vi "AlGaInPAs_ext_v00.vi"(2 "Debug Mode":bool, 3 "Elapsed Time(s)":dbl, 4 "State":enum16{"Edit", "Start", "Run", "End", "Idle"}(ring), 5 "Argument List In":string[](array[string])) -> (0 "Status Out":string, 1 "Argument List Out":string[](array[string]))   [LabVIEW 2011]
panel:
  in  "Pbub Prep":bool caption="Pre-run"
  out "Pbub Prep var":bool
  out "Pbub?":bool
  in  "Pbub Flow":dbl caption="P bubbler Flow (0-100 sccm)" format="%.2f"
  in  "Pbub Run":bool caption="Run"
  out "GAMFC3 var":dbl=100.0 caption="R3 (0-1000 sscm)" format="%.1f"
  out "GAMFC2 var":dbl=10.0 caption="R2 (0-100 sscm)" format="%.2f"
  out "GAMFC1 var":dbl caption="R1 (0-10 sscm)" format="%.2f"
  out "Ga Flow var":dbl caption="Ga Flow (0-10 sscm)" format="%.4f"
  out "In Prep var":bool
  out "Ga Prep var":bool
  out "Al Prep var":bool
  out "PH3 Prep var":bool
  out "AsH3 Prep var":bool
  out "prep_done":bool
  out "run started":bool
  out "first":bool=TRUE
  out "total time":dbl
  out "is OK?":bool
  out "AsH3?":bool
  out "PH3?":bool
  out "In?":bool
  out "Ga?":bool
  out "Al?":bool
  in  "AsH3 Prep":bool caption="Pre-run"
  in  "PH3 Prep":bool caption="Pre-run"
  in  "In Prep":bool caption="Pre-run"
  in  "prep_time":dbl caption="pre-run time (s)"
  in  "Al Prep":bool caption="Pre-run"
  in  "AsH3 Run":bool caption="Run"
  in  "AsH3 Flow":dbl caption="AsH3 Flow (0-10 sccm)" format="%.2f"
  in  "PH3 Flow":dbl caption="PH3 Flow (0-100 sccm)" format="%.2f"
  in  "PH3 Run":bool caption="Run"
  in  "In Flow":dbl caption="In Flow (0-100 sscm)" format="%.2f"
  in  "In Run":bool caption="Run"
  in  "Al Run":bool caption="Run"
  in  "Al Flow":dbl caption="Al Flow (0-100 sscm)" format="%.2f"
  in  "Cancel":bool
  in  "OK":bool
  out "tTotal(s) 2":dbl
  in  "Ga Tab Control":enum32{"Page 1", "Page 2", "Page 3"}(tab)
  in  "Ga Dilution":bool caption="Dilute"
  in  "Ga Run":bool caption="Run"
  in  "Ga Prep":bool caption="Pre-run"
  out "Ga Flow val":dbl=1.0 caption="Ga Flow (0-10 sscm)" format="%.4f"
  in  "Ga Flow set":dbl caption="Ga Flow (0-10 sscm)" format="%.4f"
  out "GAMFC1 val":dbl caption="R1 (0-10 sscm)" format="%.4f"
  out "GAMFC3 val":dbl=100.0 caption="R3 (0-1000 sscm)" format="%.1f"
  out "GAMFC2 val":dbl=10.0 caption="R2 (0-100 sscm)" format="%.2f"
  in  "GAMFC1 set":dbl=1.0 caption="R1 (0-10 sscm)" format="%.2f"
  in  "GAMFC2 set":dbl=10.0 caption="R2 (0-100 sscm)" format="%.2f"
  in  "GAMFC3 set":dbl=100.0 caption="R3 (0-1000 sscm)" format="%.1f"
  in  "Ga Calculated":u16(ring)=1 caption="Calculated" items=["Ga flow", "MFC1", "MFC2", "MFC3"]
  # "Add pre-run time to run time in editor."
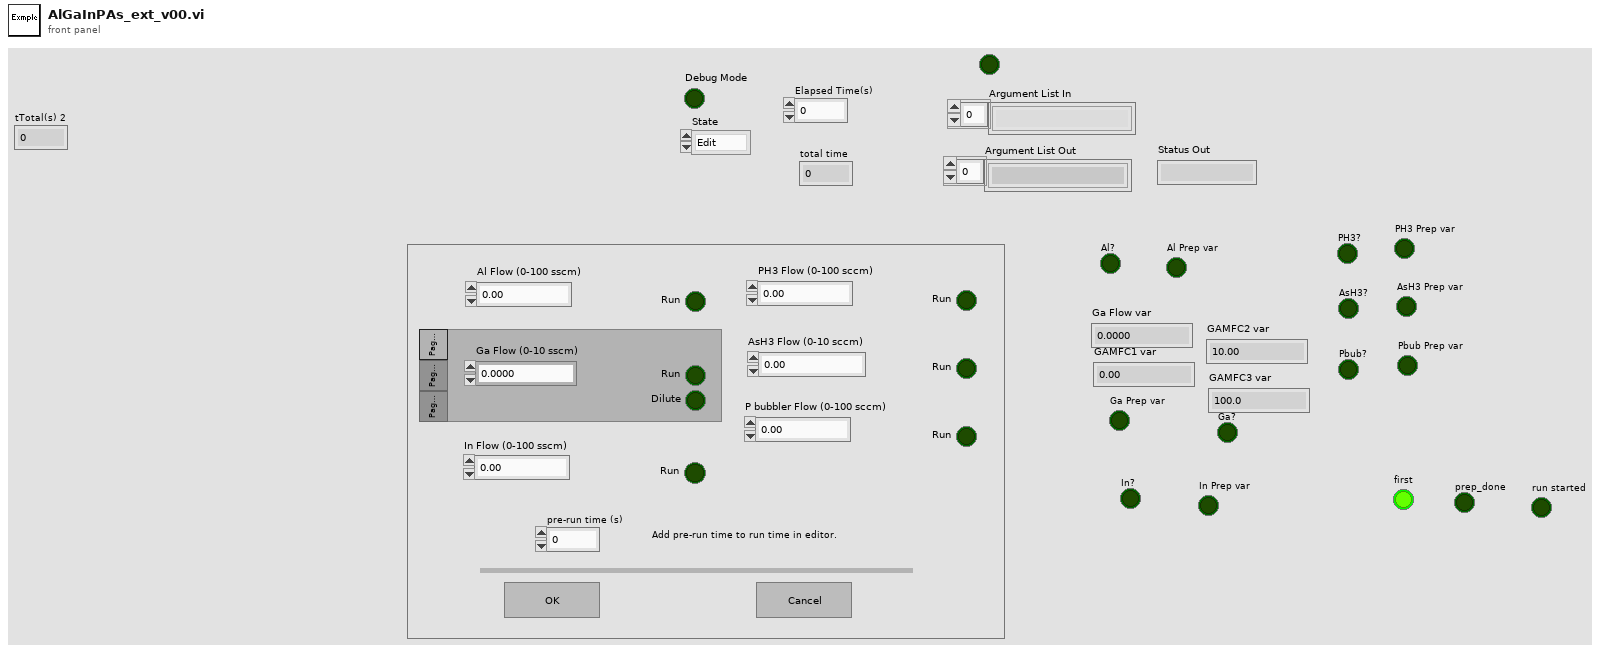
[diagram p1: front panel]
types:
  T1 = enum16{"Discrete", "Continuous", "Instantaneous", "Finite"}
  T2 = enum32{"Invalid", "Default", "Floating", "Floating/Auto-Hide", "Modal"}
  T3 = cluster{"Ga val":bool, "MFC1 val":bool, "MFC2 val":bool, "MFC3 val":bool, "Ga set":bool, "MFC1 set":bool, "MFC2 set":bool, "MFC3 set":bool}
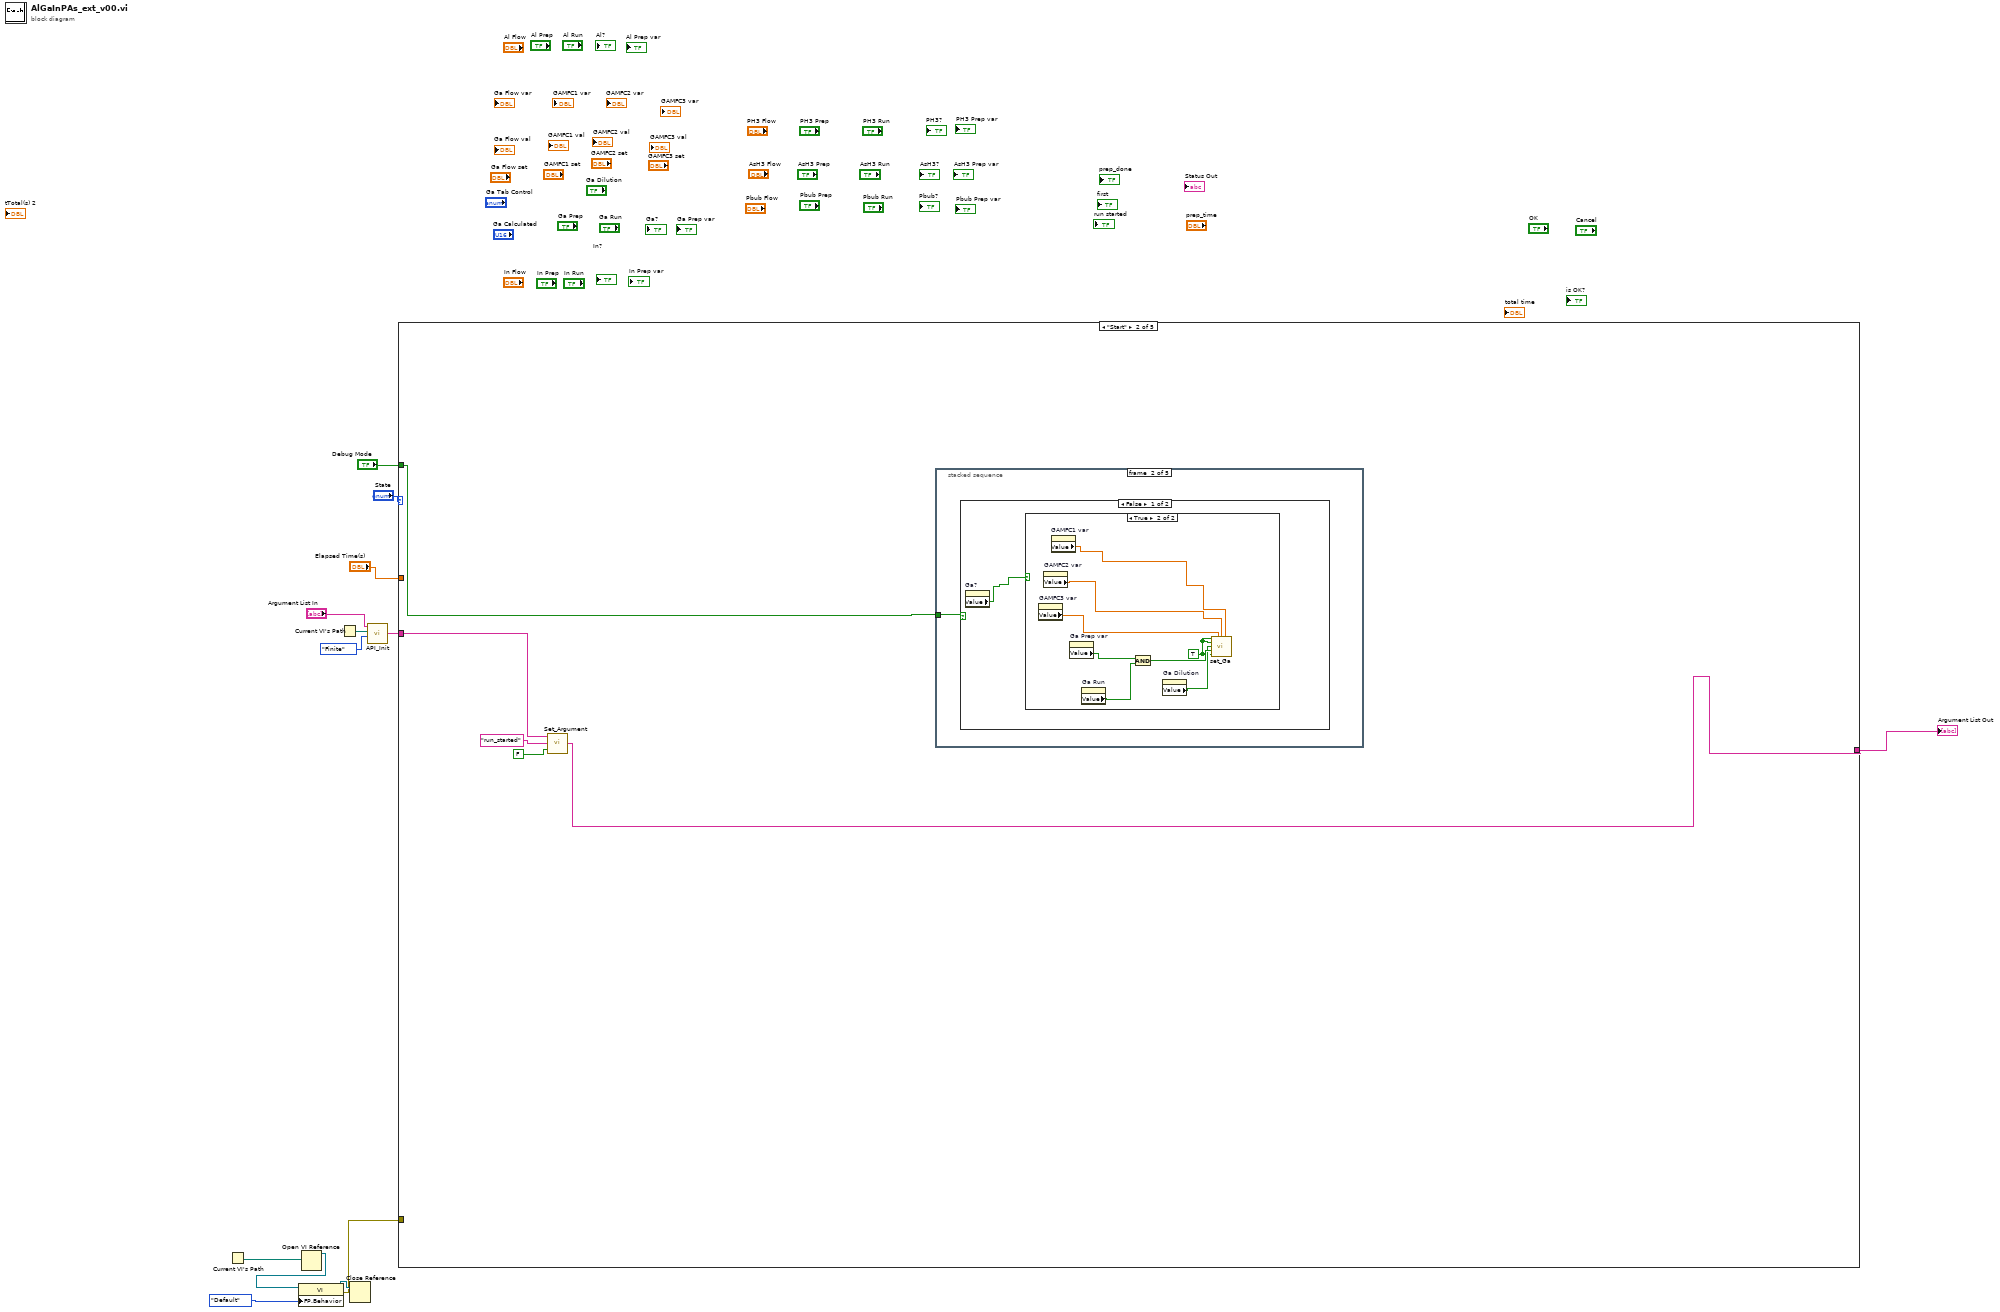
[diagram p0: block diagram]
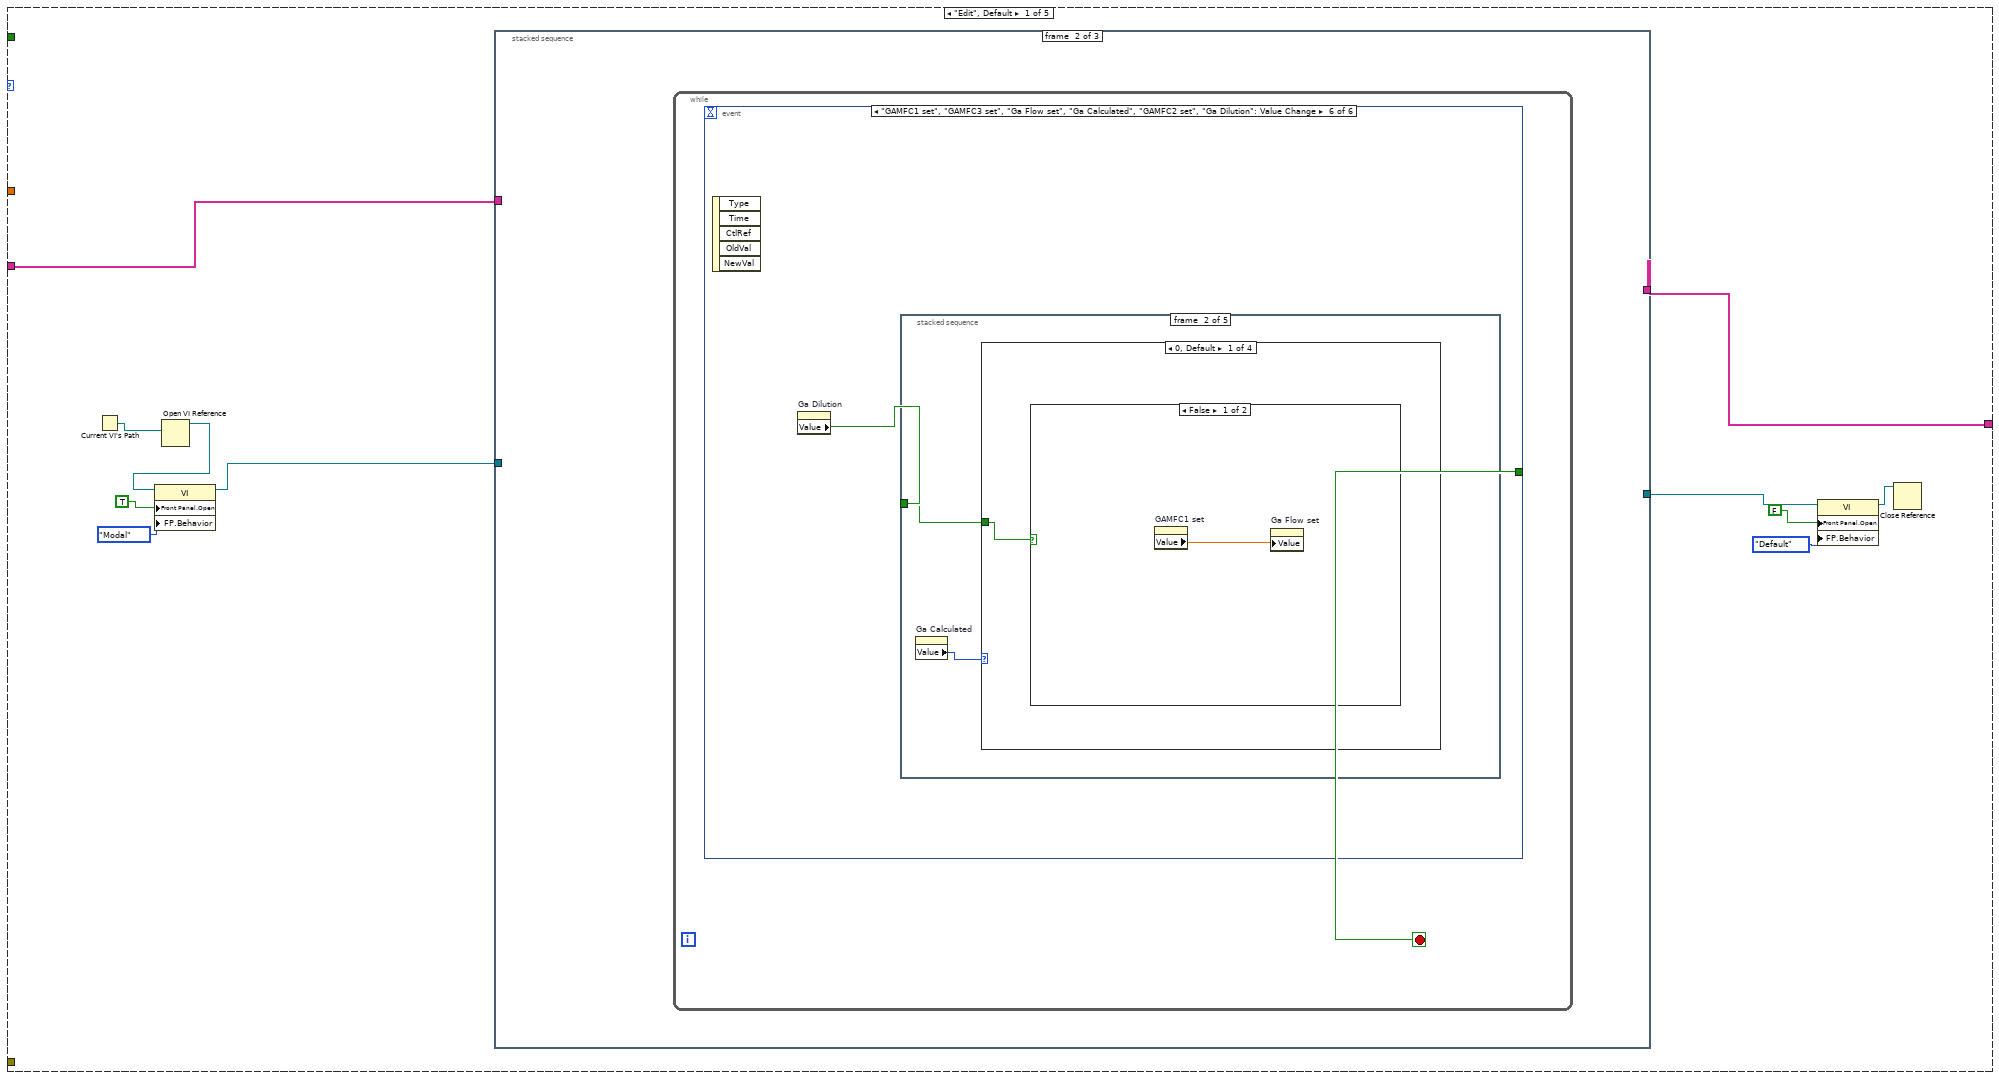
[diagram p2: hidden frame]
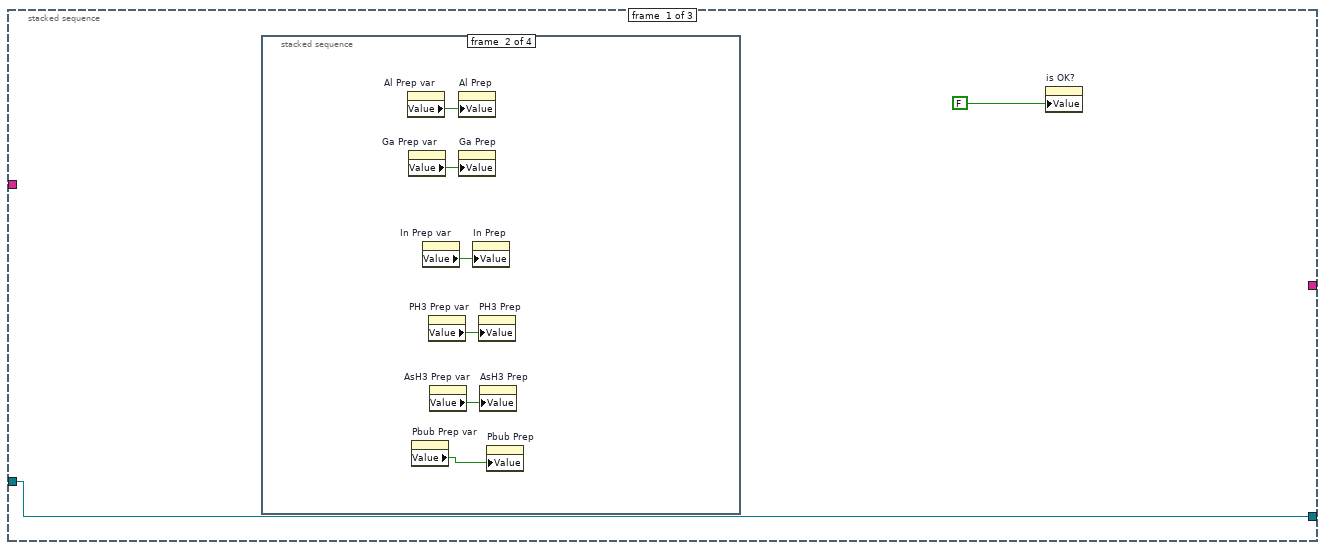
[diagram p3: hidden frame]
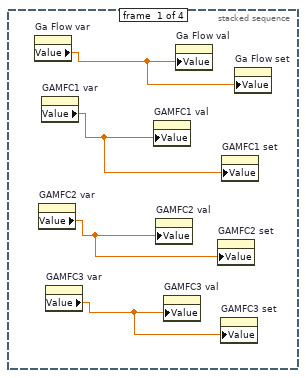
[diagram p4: hidden frame]
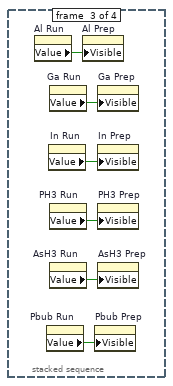
[diagram p5: hidden frame]
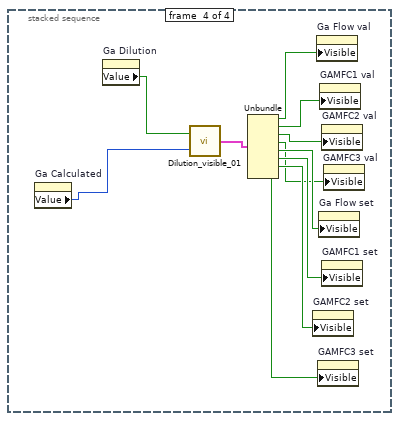
[diagram p6: hidden frame]
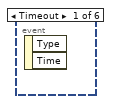
[diagram p7: hidden frame]
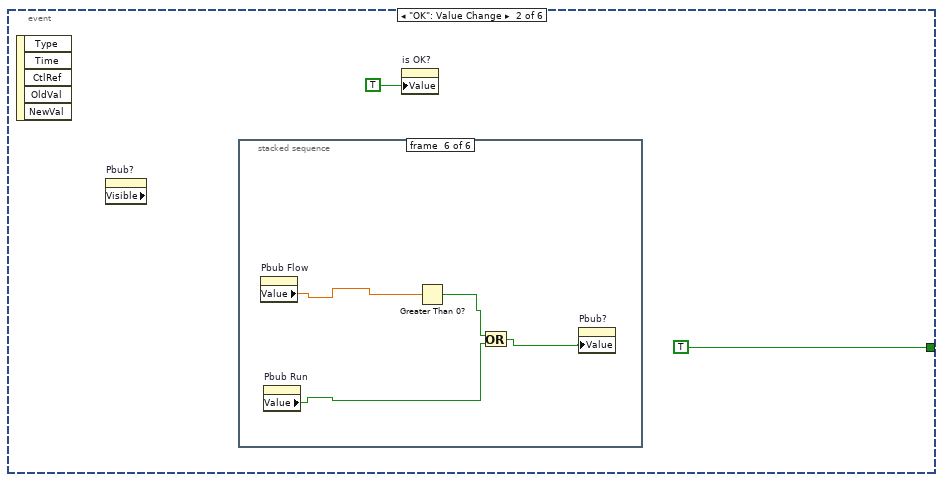
[diagram p8: hidden frame]
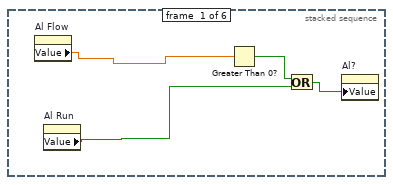
[diagram p9: hidden frame]
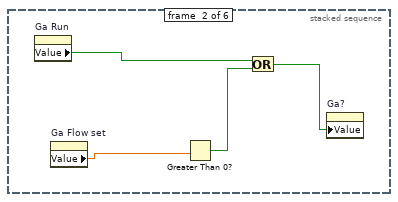
[diagram p10: hidden frame]
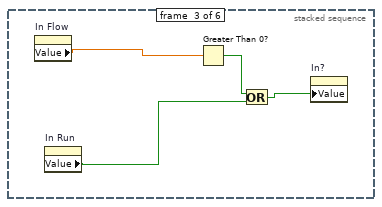
[diagram p11: hidden frame]
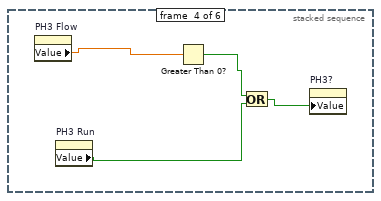
[diagram p12: hidden frame]
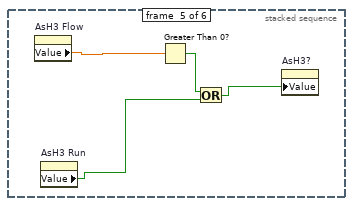
[diagram p13: hidden frame]
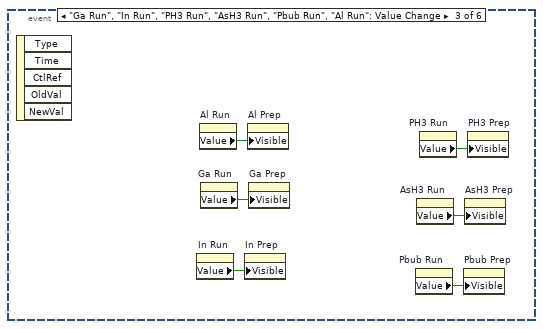
[diagram p14: hidden frame]
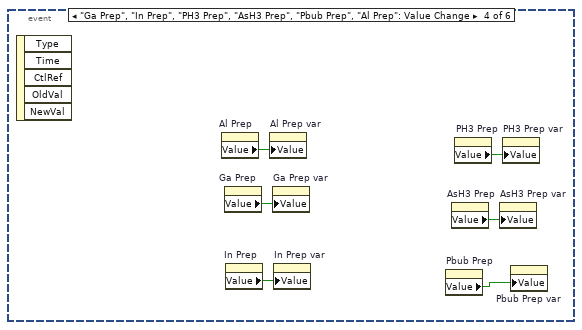
[diagram p15: hidden frame]
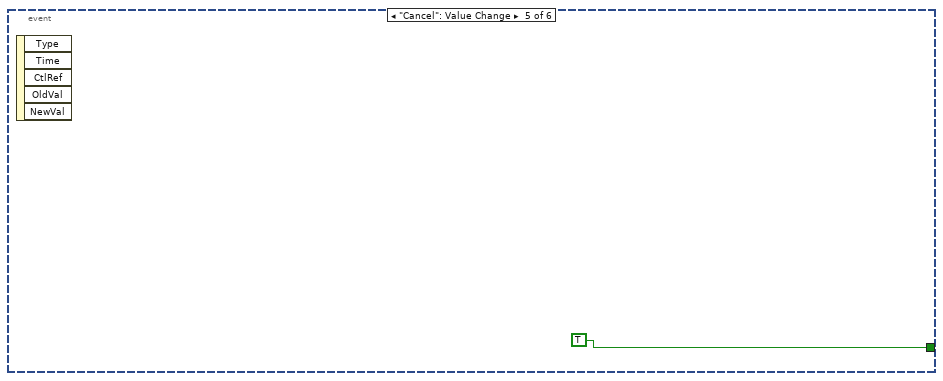
[diagram p16: hidden frame]
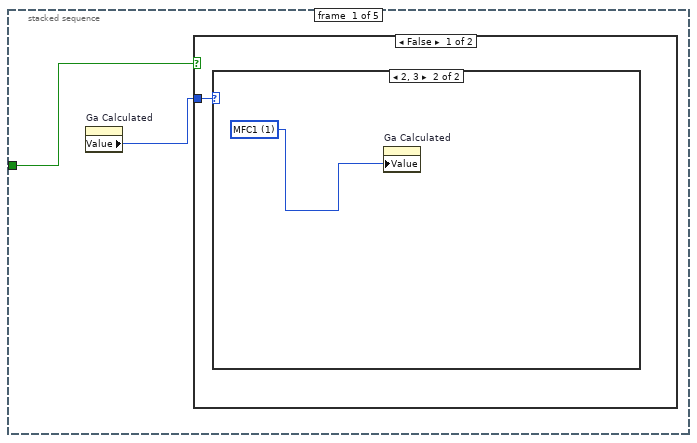
[diagram p17: hidden frame]
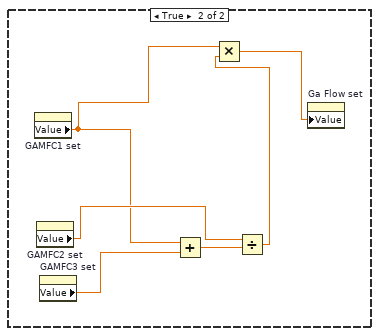
[diagram p20: hidden frame]
diagram:
  n1 = Current VI's Path() -> (path=w9:path)
  n2 = Open VI Reference(vi path=w9) -> (vi reference=w8:refnum<vi>)  [unwired: 1 in, 5 out]
  n3 = property class="VI"(reference=w8, "FP.Behavior"=T2."Default" ("Front Panel Window:Behavior")) -> (reference out=w6:refnum<vi>, error out=w5:errorcluster)  [unwired: 1 in]
  n4 = Current VI's Path() -> (path=w4:path)
  n5 = Close Reference(reference=w6) -> ()  [unwired: 1 in, 1 out]
  n6 = call "API_Init.vi"("API Mode"=T1."Finite", "VI Path"=w4, "Argument List In"="Argument List In") -> ("Argument List Out"=w1:string[])  [unwired: 1 in]
  n7 = case shown="\"Start\"" "State" {
    tunnel: "Debug Mode" -> [_ w157 w211 _ _]
    tunnel: "Elapsed Time(s)" -> [_ _ w213 _ _]
    tunnel: w1 -> [w15 w159 w210 w344 w345]
    tunnel: [w14 w158 w212 w344 w345] -> w10
    tunnel: w5 -> [_ _ _ _ _]
    frame "Edit", Default {
      n8 = Current VI's Path() -> (path=w20:path)
      n9 = Open VI Reference(vi path=w20) -> (vi reference=w19:refnum<vi>)  [unwired: 1 in, 5 out]
      n10 = property class="VI"(reference=w19, "Front Panel.Open"=TRUE ("Front Panel Window:Open"), "FP.Behavior"=T2."Modal" ("Front Panel Window:Behavior")) -> (reference out=w18:refnum<vi>)  [unwired: 1 in, 1 out]
      n11 = stacked-sequence {
        tunnel: w15 -> [_ _ w152]
        tunnel: w18 -> [w26 _ _]
        tunnel: [w26 _ _] -> w22
        tunnel: [_ _ w150] -> w14
        frame #0 {
          n12 = stacked-sequence {
            frame #0 {
              n13 = property on="Ga Flow var" class="DigNum (strict)"() -> ("Value"=w30:dbl)  [unwired: 2 in, 2 out]
              n14 = property on="GAMFC2 var" class="DigNum (strict)"() -> ("Value"=w28:dbl)  [unwired: 2 in, 2 out]
              n15 = property on="GAMFC1 var" class="DigNum (strict)"() -> ("Value"=w27:dbl)  [unwired: 2 in, 2 out]
              n16 = property on="GAMFC3 var" class="DigNum (strict)"() -> ("Value"=w29:dbl)  [unwired: 2 in, 2 out]
              n17 = property on="GAMFC1 val" class="DigNum (strict)"("Value"=w27) -> ()  [unwired: 2 in, 2 out]
              n18 = property on="GAMFC2 val" class="DigNum (strict)"("Value"=w28) -> ()  [unwired: 2 in, 2 out]
              n19 = property on="GAMFC3 val" class="DigNum (strict)"("Value"=w29) -> ()  [unwired: 2 in, 2 out]
              n20 = property on="Ga Flow val" class="DigNum (strict)"("Value"=w30) -> ()  [unwired: 2 in, 2 out]
              n21 = property on="GAMFC2 set" class="DigNum (strict)"("Value"=w28) -> ()  [unwired: 2 in, 2 out]
              n22 = property on="GAMFC3 set" class="DigNum (strict)"("Value"=w29) -> ()  [unwired: 2 in, 2 out]
              n23 = property on="GAMFC1 set" class="DigNum (strict)"("Value"=w27) -> ()  [unwired: 2 in, 2 out]
              n24 = property on="Ga Flow set" class="DigNum (strict)"("Value"=w30) -> ()  [unwired: 2 in, 2 out]
            }
            frame #1 {
              n25 = property on="Al Prep var" class="Bool (strict)"() -> ("Value"=w36:bool)  [unwired: 2 in, 2 out]
              n26 = property on="Ga Prep var" class="Bool (strict)"() -> ("Value"=w35:bool)  [unwired: 2 in, 2 out]
              n27 = property on="Pbub Prep var" class="Bool (strict)"() -> ("Value"=w31:bool)  [unwired: 2 in, 2 out]
              n28 = property on="In Prep var" class="Bool (strict)"() -> ("Value"=w34:bool)  [unwired: 2 in, 2 out]
              n29 = property on="PH3 Prep var" class="Bool (strict)"() -> ("Value"=w33:bool)  [unwired: 2 in, 2 out]
              n30 = property on="AsH3 Prep var" class="Bool (strict)"() -> ("Value"=w32:bool)  [unwired: 2 in, 2 out]
              n31 = property on="Al Prep" class="Bool (strict)"("Value"=w36) -> ()  [unwired: 2 in, 2 out]
              n32 = property on="Ga Prep" class="Bool (strict)"("Value"=w35) -> ()  [unwired: 2 in, 2 out]
              n33 = property on="In Prep" class="Bool (strict)"("Value"=w34) -> ()  [unwired: 2 in, 2 out]
              n34 = property on="PH3 Prep" class="Bool (strict)"("Value"=w33) -> ()  [unwired: 2 in, 2 out]
              n35 = property on="AsH3 Prep" class="Bool (strict)"("Value"=w32) -> ()  [unwired: 2 in, 2 out]
              n36 = property on="Pbub Prep" class="Bool (strict)"("Value"=w31) -> ()  [unwired: 2 in, 2 out]
            }
            frame #2 {
              n37 = property on="Al Run" class="Bool (strict)"() -> ("Value"=w42:bool)  [unwired: 2 in, 2 out]
              n38 = property on="Pbub Run" class="Bool (strict)"() -> ("Value"=w37:bool)  [unwired: 2 in, 2 out]
              n39 = property on="In Run" class="Bool (strict)"() -> ("Value"=w40:bool)  [unwired: 2 in, 2 out]
              n40 = property on="Ga Run" class="Bool (strict)"() -> ("Value"=w41:bool)  [unwired: 2 in, 2 out]
              n41 = property on="PH3 Run" class="Bool (strict)"() -> ("Value"=w39:bool)  [unwired: 2 in, 2 out]
              n42 = property on="AsH3 Run" class="Bool (strict)"() -> ("Value"=w38:bool)  [unwired: 2 in, 2 out]
              n43 = property on="Al Prep" class="Bool (strict)"("Visible"=w42) -> ()  [unwired: 2 in, 2 out]
              n44 = property on="Pbub Prep" class="Bool (strict)"("Visible"=w37) -> ()  [unwired: 2 in, 2 out]
              n45 = property on="Ga Prep" class="Bool (strict)"("Visible"=w41) -> ()  [unwired: 2 in, 2 out]
              n46 = property on="In Prep" class="Bool (strict)"("Visible"=w40) -> ()  [unwired: 2 in, 2 out]
              n47 = property on="PH3 Prep" class="Bool (strict)"("Visible"=w39) -> ()  [unwired: 2 in, 2 out]
              n48 = property on="AsH3 Prep" class="Bool (strict)"("Visible"=w38) -> ()  [unwired: 2 in, 2 out]
            }
            frame #3 {
              n49 = property on="Ga Calculated" class="Ring (strict)"() -> ("Value"=w43:u16)  [unwired: 2 in, 2 out]
              n50 = property on="Ga Dilution" class="Bool (strict)"() -> ("Value"=w53:bool)  [unwired: 2 in, 2 out]
              n51 = call "Dilution_visible_01.vi"("calculated"=w43, "dilution"=w53) -> ("Visible"=w45:T3)
              n52 = Unbundle(w45) -> ("Ga val"=w46:bool, "MFC1 val"=w47:bool, "MFC2 val"=w44:bool, "MFC3 val"=w48:bool, "Ga set"=w49:bool, "MFC1 set"=w50:bool, "MFC2 set"=w51:bool, "MFC3 set"=w52:bool)
              n53 = property on="GAMFC2 set" class="DigNum (strict)"("Visible"=w51) -> ()  [unwired: 2 in, 2 out]
              n54 = property on="Ga Flow val" class="DigNum (strict)"("Visible"=w46) -> ()  [unwired: 2 in, 2 out]
              n55 = property on="GAMFC3 set" class="DigNum (strict)"("Visible"=w52) -> ()  [unwired: 2 in, 2 out]
              n56 = property on="Ga Flow set" class="DigNum (strict)"("Visible"=w49) -> ()  [unwired: 2 in, 2 out]
              n57 = property on="GAMFC1 val" class="DigNum (strict)"("Visible"=w47) -> ()  [unwired: 2 in, 2 out]
              n58 = property on="GAMFC2 val" class="DigNum (strict)"("Visible"=w44) -> ()  [unwired: 2 in, 2 out]
              n59 = property on="GAMFC1 set" class="DigNum (strict)"("Visible"=w50) -> ()  [unwired: 2 in, 2 out]
              n60 = property on="GAMFC3 val" class="DigNum (strict)"("Visible"=w48) -> ()  [unwired: 2 in, 2 out]
            }
          }
          n61 = property on="is OK?" class="Bool (strict)"("Value"=FALSE ("is OK?")) -> ()  [unwired: 2 in, 2 out]
        }
        frame #1 {
          n62 = while {
            stop <- w54 stop-if-true
            n63 = event shown="[5] \"GAMFC1 set\", \"GAMFC3 set\", \"Ga Flow set\", \"Ga Calculated\", \"GAMFC2 set\", \"Ga Dilution\": Value Change" {
              selector: _ -> [_ _ _ _ _ _]
              dyn-events: _ -> [_ _ _ _ _ _]
              timeout: _ -> [_ _ _ _ _ _]
              tunnel: [_ TRUE _ _ TRUE _] -> w54
              event Timeout {
                n64 = event-data() -> ()  [unwired: 1 in, 2 out]
              }
              event "OK": Value Change {
                n65 = event-data() -> ()  [unwired: 1 in, 5 out]
                n66 = property on="Pbub?" class="Bool (strict)" props=["Visible"]() -> ()  [unwired: 2 in, 3 out]
                n67 = stacked-sequence {
                  frame #0 {
                    n68 = property on="Al Flow" class="DigNum (strict)"() -> ("Value"=w59:dbl)  [unwired: 2 in, 2 out]
                    n69 = property on="Al Run" class="Bool (strict)"() -> ("Value"=w58:bool)  [unwired: 2 in, 2 out]
                    n70 = Greater Than 0?(x=w59) -> (x > 0?=w60:bool)
                    n71 = Or(x=w60, y=w58) -> (x .or. y?=w57:bool)
                    n72 = property on="Al?" class="Bool (strict)"("Value"=w57) -> ()  [unwired: 2 in, 2 out]
                  }
                  frame #1 {
                    n73 = property on="Ga Run" class="Bool (strict)"() -> ("Value"=w62:bool)  [unwired: 2 in, 2 out]
                    n74 = property on="Ga Flow set" class="DigNum (strict)"() -> ("Value"=w63:dbl)  [unwired: 2 in, 2 out]
                    n75 = Greater Than 0?(x=w63) -> (x > 0?=w64:bool)
                    n76 = Or(x=w62, y=w64) -> (x .or. y?=w61:bool)
                    n77 = property on="Ga?" class="Bool (strict)"("Value"=w61) -> ()  [unwired: 2 in, 2 out]
                  }
                  frame #2 {
                    n78 = property on="In Flow" class="DigNum (strict)"() -> ("Value"=w66:dbl)  [unwired: 2 in, 2 out]
                    n79 = property on="In Run" class="Bool (strict)"() -> ("Value"=w67:bool)  [unwired: 2 in, 2 out]
                    n80 = Greater Than 0?(x=w66) -> (x > 0?=w68:bool)
                    n81 = Or(x=w68, y=w67) -> (x .or. y?=w65:bool)
                    n82 = property on="In?" class="Bool (strict)"("Value"=w65) -> ()  [unwired: 2 in, 2 out]
                  }
                  frame #3 {
                    n83 = property on="PH3 Flow" class="DigNum (strict)"() -> ("Value"=w71:dbl)  [unwired: 2 in, 2 out]
                    n84 = property on="PH3 Run" class="Bool (strict)"() -> ("Value"=w70:bool)  [unwired: 2 in, 2 out]
                    n85 = Greater Than 0?(x=w71) -> (x > 0?=w72:bool)
                    n86 = Or(x=w72, y=w70) -> (x .or. y?=w69:bool)
                    n87 = property on="PH3?" class="Bool (strict)"("Value"=w69) -> ()  [unwired: 2 in, 2 out]
                  }
                  frame #4 {
                    n88 = property on="AsH3 Flow" class="DigNum (strict)"() -> ("Value"=w75:dbl)  [unwired: 2 in, 2 out]
                    n89 = property on="AsH3 Run" class="Bool (strict)"() -> ("Value"=w74:bool)  [unwired: 2 in, 2 out]
                    n90 = Greater Than 0?(x=w75) -> (x > 0?=w76:bool)
                    n91 = Or(x=w76, y=w74) -> (x .or. y?=w73:bool)
                    n92 = property on="AsH3?" class="Bool (strict)"("Value"=w73) -> ()  [unwired: 2 in, 2 out]
                  }
                  frame #5 {
                    n93 = property on="Pbub Flow" class="DigNum (strict)"() -> ("Value"=w78:dbl)  [unwired: 2 in, 2 out]
                    n94 = property on="Pbub Run" class="Bool (strict)"() -> ("Value"=w77:bool)  [unwired: 2 in, 2 out]
                    n95 = Greater Than 0?(x=w78) -> (x > 0?=w80:bool)
                    n96 = Or(x=w80, y=w77) -> (x .or. y?=w79:bool)
                    n97 = property on="Pbub?" class="Bool (strict)"("Value"=w79) -> ()  [unwired: 2 in, 2 out]
                  }
                }
                n98 = property on="is OK?" class="Bool (strict)"("Value"=TRUE ("is OK?")) -> ()  [unwired: 2 in, 2 out]
              }
              event "Ga Run", "In Run", "PH3 Run", "AsH3 Run", "Pbub Run", "Al Run": Value Change {
                n99 = event-data() -> ()  [unwired: 1 in, 5 out]
                n100 = property on="In Run" class="Bool (strict)"() -> ("Value"=w84:bool)  [unwired: 2 in, 2 out]
                n101 = property on="Al Run" class="Bool (strict)"() -> ("Value"=w86:bool)  [unwired: 2 in, 2 out]
                n102 = property on="Ga Run" class="Bool (strict)"() -> ("Value"=w85:bool)  [unwired: 2 in, 2 out]
                n103 = property on="In Prep" class="Bool (strict)"("Visible"=w84) -> ()  [unwired: 2 in, 2 out]
                n104 = property on="Al Prep" class="Bool (strict)"("Visible"=w86) -> ()  [unwired: 2 in, 2 out]
                n105 = property on="Ga Prep" class="Bool (strict)"("Visible"=w85) -> ()  [unwired: 2 in, 2 out]
                n106 = property on="Pbub Run" class="Bool (strict)"() -> ("Value"=w81:bool)  [unwired: 2 in, 2 out]
                n107 = property on="AsH3 Run" class="Bool (strict)"() -> ("Value"=w83:bool)  [unwired: 2 in, 2 out]
                n108 = property on="PH3 Run" class="Bool (strict)"() -> ("Value"=w82:bool)  [unwired: 2 in, 2 out]
                n109 = property on="Pbub Prep" class="Bool (strict)"("Visible"=w81) -> ()  [unwired: 2 in, 2 out]
                n110 = property on="AsH3 Prep" class="Bool (strict)"("Visible"=w83) -> ()  [unwired: 2 in, 2 out]
                n111 = property on="PH3 Prep" class="Bool (strict)"("Visible"=w82) -> ()  [unwired: 2 in, 2 out]
              }
              event "Ga Prep", "In Prep", "PH3 Prep", "AsH3 Prep", "Pbub Prep", "Al Prep": Value Change {
                n112 = event-data() -> ()  [unwired: 1 in, 5 out]
                n113 = property on="Al Prep" class="Bool (strict)"() -> ("Value"=w92:bool)  [unwired: 2 in, 2 out]
                n114 = property on="Ga Prep" class="Bool (strict)"() -> ("Value"=w91:bool)  [unwired: 2 in, 2 out]
                n115 = property on="In Prep" class="Bool (strict)"() -> ("Value"=w90:bool)  [unwired: 2 in, 2 out]
                n116 = property on="Al Prep var" class="Bool (strict)"("Value"=w92) -> ()  [unwired: 2 in, 2 out]
                n117 = property on="Ga Prep var" class="Bool (strict)"("Value"=w91) -> ()  [unwired: 2 in, 2 out]
                n118 = property on="In Prep var" class="Bool (strict)"("Value"=w90) -> ()  [unwired: 2 in, 2 out]
                n119 = property on="Pbub Prep" class="Bool (strict)"() -> ("Value"=w87:bool)  [unwired: 2 in, 2 out]
                n120 = property on="AsH3 Prep" class="Bool (strict)"() -> ("Value"=w88:bool)  [unwired: 2 in, 2 out]
                n121 = property on="PH3 Prep" class="Bool (strict)"() -> ("Value"=w89:bool)  [unwired: 2 in, 2 out]
                n122 = property on="AsH3 Prep var" class="Bool (strict)"("Value"=w88) -> ()  [unwired: 2 in, 2 out]
                n123 = property on="PH3 Prep var" class="Bool (strict)"("Value"=w89) -> ()  [unwired: 2 in, 2 out]
                n124 = property on="Pbub Prep var" class="Bool (strict)"("Value"=w87) -> ()  [unwired: 2 in, 2 out]
              }
              event "Cancel": Value Change {
                n125 = event-data() -> ()  [unwired: 1 in, 5 out]
              }
              event "GAMFC1 set", "GAMFC3 set", "Ga Flow set", "Ga Calculated", "GAMFC2 set", "Ga Dilution": Value Change {
                n126 = event-data() -> ()  [unwired: 1 in, 5 out]
                n127 = property on="Ga Dilution" class="Bool (strict)"() -> ("Value"=w94:bool)  [unwired: 2 in, 2 out]
                n128 = stacked-sequence {
                  tunnel: w94 -> [w96 w100 w141 _ w146]
                  frame #0 {
                    n129 = property on="Ga Calculated" class="Ring (strict)"() -> ("Value"=w95:u16)  [unwired: 2 in, 2 out]
                    n130 = case shown="False" w96 {
                      tunnel: w95 -> [w97 _]
                      frame False {
                        n131 = case shown="2, 3" w97 {
                          frame 0, 1, Default {
                          }
                          frame 2, 3 {
                            w98 = u16 1 items=["Ga flow", "MFC1", "MFC2", "MFC3"] ("Ga calculated")
                            n132 = property on="Ga Calculated" class="Ring (strict)"("Value"=w98) -> ()  [unwired: 2 in, 2 out]
                          }
                        }
                      }
                      frame True {
                      }
                    }
                  }
                  frame #1 {
                    n133 = property on="Ga Calculated" class="Ring (strict)"() -> ("Value"=w99:u16)  [unwired: 2 in, 2 out]
                    n134 = case shown="0, Default" w99 {
                      tunnel: w100 -> [w101 w109 w117 w124]
                      frame 0, Default {
                        n135 = case shown="False" w101 {
                          frame False {
                            n136 = property on="GAMFC1 set" class="DigNum (strict)"() -> ("Value"=w102:dbl)  [unwired: 2 in, 2 out]
                            n137 = property on="Ga Flow set" class="DigNum (strict)"("Value"=w102) -> ()  [unwired: 2 in, 2 out]
                          }
                          frame True {
                            n138 = property on="GAMFC1 set" class="DigNum (strict)"() -> ("Value"=w104:dbl)  [unwired: 2 in, 2 out]
                            n139 = property on="GAMFC2 set" class="DigNum (strict)"() -> ("Value"=w106:dbl)  [unwired: 2 in, 2 out]
                            n140 = property on="GAMFC3 set" class="DigNum (strict)"() -> ("Value"=w108:dbl)  [unwired: 2 in, 2 out]
                            n141 = Add(x=w104, y=w108) -> (x+y=w107:dbl)
                            n142 = Divide(x=w106, y=w107) -> (x/y=w105:dbl)
                            n143 = Multiply(x=w104, y=w105) -> (x*y=w103:dbl)
                            n144 = property on="Ga Flow set" class="DigNum (strict)"("Value"=w103) -> ()  [unwired: 2 in, 2 out]
                          }
                        }
                      }
                      frame 1 {
                        n145 = case shown="True" w109 {
                          frame False {
                            n146 = property on="Ga Flow set" class="DigNum (strict)"() -> ("Value"=w110:dbl)  [unwired: 2 in, 2 out]
                            n147 = property on="GAMFC1 set" class="DigNum (strict)"("Value"=w110) -> ()  [unwired: 2 in, 2 out]
                          }
                          frame True {
                            n148 = property on="Ga Flow set" class="DigNum (strict)"() -> ("Value"=w115:dbl)  [unwired: 2 in, 2 out]
                            n149 = property on="GAMFC2 set" class="DigNum (strict)"() -> ("Value"=w116:dbl)  [unwired: 2 in, 2 out]
                            n150 = property on="GAMFC3 set" class="DigNum (strict)"() -> ("Value"=w114:dbl)  [unwired: 2 in, 2 out]
                            n151 = Subtract(x=w116, y=w115) -> (x-y=w112:dbl)
                            n152 = Multiply(x=w115, y=w114) -> (x*y=w113:dbl)
                            n153 = Divide(x=w113, y=w112) -> (x/y=w111:dbl)
                            n154 = property on="GAMFC1 set" class="DigNum (strict)"("Value"=w111) -> ()  [unwired: 2 in, 2 out]
                          }
                        }
                      }
                      frame 2 {
                        n155 = case shown="True" w117 {
                          frame False {
                          }
                          frame True {
                            n156 = property on="GAMFC1 set" class="DigNum (strict)"() -> ("Value"=w119:dbl)  [unwired: 2 in, 2 out]
                            n157 = property on="GAMFC3 set" class="DigNum (strict)"() -> ("Value"=w121:dbl)  [unwired: 2 in, 2 out]
                            n158 = property on="Ga Flow set" class="DigNum (strict)"() -> ("Value"=w122:dbl)  [unwired: 2 in, 2 out]
                            n159 = Add(x=w119, y=w121) -> (x+y=w123:dbl)
                            n160 = Multiply(x=w122, y=w123) -> (x*y=w120:dbl)
                            n161 = Divide(x=w120, y=w119) -> (x/y=w118:dbl)
                            n162 = property on="GAMFC2 set" class="DigNum (strict)"("Value"=w118) -> ()  [unwired: 2 in, 2 out]
                          }
                        }
                      }
                      frame 3 {
                        n163 = case shown="True" w124 {
                          frame False {
                          }
                          frame True {
                            n164 = property on="GAMFC2 set" class="DigNum (strict)"() -> ("Value"=w130:dbl)  [unwired: 2 in, 2 out]
                            n165 = property on="Ga Flow set" class="DigNum (strict)"() -> ("Value"=w128:dbl)  [unwired: 2 in, 2 out]
                            n166 = property on="GAMFC1 set" class="DigNum (strict)"() -> ("Value"=w129:dbl)  [unwired: 2 in, 2 out]
                            n167 = Subtract(x=w130, y=w128) -> (x-y=w126:dbl)
                            n168 = Divide(x=w129, y=w128) -> (x/y=w127:dbl)
                            n169 = Multiply(x=w127, y=w126) -> (x*y=w125:dbl)
                            n170 = property on="GAMFC3 set" class="DigNum (strict)"("Value"=w125) -> ()  [unwired: 2 in, 2 out]
                          }
                        }
                      }
                    }
                  }
                  frame #2 {
                    n171 = property on="Ga Calculated" class="Ring (strict)"() -> ("Value"=w131:u16)  [unwired: 2 in, 2 out]
                    n172 = call "Dilution_visible_01.vi"("calculated"=w131, "dilution"=w141) -> ("Visible"=w137:T3)
                    n173 = Unbundle(w137) -> ("Ga val"=w140:bool, "MFC1 val"=w139:bool, "MFC2 val"=w138:bool, "MFC3 val"=w136:bool, "Ga set"=w135:bool, "MFC1 set"=w134:bool, "MFC2 set"=w133:bool, "MFC3 set"=w132:bool)
                    n174 = property on="Ga Flow set" class="DigNum (strict)"("Visible"=w135) -> ()  [unwired: 2 in, 2 out]
                    n175 = property on="GAMFC1 set" class="DigNum (strict)"("Visible"=w134) -> ()  [unwired: 2 in, 2 out]
                    n176 = property on="GAMFC3 set" class="DigNum (strict)"("Visible"=w132) -> ()  [unwired: 2 in, 2 out]
                    n177 = property on="GAMFC2 set" class="DigNum (strict)"("Visible"=w133) -> ()  [unwired: 2 in, 2 out]
                    n178 = property on="Ga Flow val" class="DigNum (strict)"("Visible"=w140) -> ()  [unwired: 2 in, 2 out]
                    n179 = property on="GAMFC1 val" class="DigNum (strict)"("Visible"=w139) -> ()  [unwired: 2 in, 2 out]
                    n180 = property on="GAMFC2 val" class="DigNum (strict)"("Visible"=w138) -> ()  [unwired: 2 in, 2 out]
                    n181 = property on="GAMFC3 val" class="DigNum (strict)"("Visible"=w136) -> ()  [unwired: 2 in, 2 out]
                  }
                  frame #3 {
                    n182 = property on="GAMFC1 set" class="DigNum (strict)"() -> ("Value"=w144:dbl)  [unwired: 2 in, 2 out]
                    n183 = property on="Ga Flow set" class="DigNum (strict)"() -> ("Value"=w145:dbl)  [unwired: 2 in, 2 out]
                    n184 = property on="GAMFC2 set" class="DigNum (strict)"() -> ("Value"=w143:dbl)  [unwired: 2 in, 2 out]
                    n185 = property on="GAMFC3 set" class="DigNum (strict)"() -> ("Value"=w142:dbl)  [unwired: 2 in, 2 out]
                    n186 = property on="GAMFC3 val" class="DigNum (strict)"("Value"=w142) -> ()  [unwired: 2 in, 2 out]
                    n187 = property on="GAMFC1 val" class="DigNum (strict)"("Value"=w144) -> ()  [unwired: 2 in, 2 out]
                    n188 = property on="GAMFC2 val" class="DigNum (strict)"("Value"=w143) -> ()  [unwired: 2 in, 2 out]
                    n189 = property on="Ga Flow val" class="DigNum (strict)"("Value"=w145) -> ()  [unwired: 2 in, 2 out]
                    n190 = property on="GAMFC3 var" class="DigNum (strict)"("Value"=w142) -> ()  [unwired: 2 in, 2 out]
                    n191 = property on="GAMFC1 var" class="DigNum (strict)"("Value"=w144) -> ()  [unwired: 2 in, 2 out]
                    n192 = property on="GAMFC2 var" class="DigNum (strict)"("Value"=w143) -> ()  [unwired: 2 in, 2 out]
                    n193 = property on="Ga Flow var" class="DigNum (strict)"("Value"=w145) -> ()  [unwired: 2 in, 2 out]
                  }
                  frame #4 {
                    n194 = case shown="True" w146 {
                      frame False {
                        n195 = property on="Ga Calculated" class="Ring (strict)"("Disabled Items []"=i32[] [2, 3]) -> ()  [unwired: 2 in, 2 out]
                      }
                      frame True {
                        n196 = property on="Ga Calculated" class="Ring (strict)"("Disabled Items []"=i32[] []) -> ()  [unwired: 2 in, 2 out]
                      }
                    }
                  }
                }
              }
            }
          }
        }
        frame #2 {
          n197 = property on="is OK?" class="Bool (strict)"() -> ("Value"=w149:bool)  [unwired: 2 in, 2 out]
          n198 = case shown="True" w149 {
            tunnel: w152 -> [w155 w156]
            tunnel: [w155 w156] -> w151
            frame False {
            }
            frame True {
            }
          }
          n199 = Not(x=w149) -> (.not. x?=w154:bool)
          n200 = Current VI's Path() -> (path=w153:path)
          n201 = call "API_Edit.vi"("Cancel"=w154, "OK"=w149, "VI Path"=w153, "Argument List In"=w151) -> ("Argument List Out"=w150:string[])
        }
      }
      n202 = property class="VI"(reference=w22, "Front Panel.Open"=FALSE ("Front Panel Window:Open"), "FP.Behavior"=T2."Default" ("Front Panel Window:Behavior")) -> (reference out=w23:refnum<vi>)  [unwired: 1 in, 1 out]
      n203 = Close Reference(reference=w23) -> ()  [unwired: 1 in, 1 out]
    }
    frame "Start" {
      n204 = call "Set_Argument.vi"("Enable"=FALSE, "Argument"="run_started", "Argument List In"=w159) -> ("Argument List Out"=w158:string[])
      n205 = stacked-sequence {
        tunnel: w157 -> [w162 w171 w183 w192 w201]
        frame #0 {
          n206 = case shown="False" w162 {
            frame False {
              n207 = property on="Al?" class="Bool (strict)"() -> ("Value"=w163:bool)  [unwired: 2 in, 2 out]
              n208 = case shown="True" w163 {
                frame False {
                  w164 = FALSE ("Al Active")
                  n209 = call "set_Al.vi"("Aluminum Flow"=0.0, "Al Remote"=w164, "Al Run"=w164, "Al Bubbler"=w164, "Al Active"=w164) -> ()  [unwired: 5 out]
                }
                frame True {
                  w170 = TRUE ("Al Active")
                  n210 = property on="Al Prep" class="Bool (strict)"() -> ("Value"=w168:bool)  [unwired: 2 in, 2 out]
                  n211 = property on="Al Run" class="Bool (strict)"() -> ("Value"=w167:bool)  [unwired: 2 in, 2 out]
                  n212 = property on="Al Flow" class="DigNum (strict)"() -> ("Value"=w169:dbl)  [unwired: 2 in, 2 out]
                  n213 = And(x=w168, y=w167) -> (x .and. y?=w166:bool)
                  n214 = call "set_Al.vi"("Aluminum Flow"=w169, "Al Run"=w166, "Al Bubbler"=w170, "Al Active"=w170) -> ()  [unwired: 1 in, 5 out]
                }
              }
            }
            frame True {
            }
          }
        }
        frame #1 {
          n215 = case shown="False" w171 {
            frame False {
              n216 = property on="Ga?" class="Bool (strict)"() -> ("Value"=w172:bool)  [unwired: 2 in, 2 out]
              n217 = case shown="True" w172 {
                frame False {
                  w174 = FALSE ("Ga Active")
                  w173 = 0.0 ("Ga Flow 1")
                  n218 = call "set_Ga.vi"("Ga Active"=w174, "Ga Flow 3"=w173, "Ga Flow 2"=w173, "Ga Flow 1"=w173, "Ga Bubbler"=w174, "Ga H2 Dilute"=w174, "Ga Run"=w174, "Ga Remote"=w174) -> ()  [unwired: 8 out]
                }
                frame True {
                  w178 = TRUE ("Ga Active")
                  n219 = property on="GAMFC3 var" class="DigNum (strict)"() -> ("Value"=w175:dbl)  [unwired: 2 in, 2 out]
                  n220 = property on="GAMFC2 var" class="DigNum (strict)"() -> ("Value"=w176:dbl)  [unwired: 2 in, 2 out]
                  n221 = property on="GAMFC1 var" class="DigNum (strict)"() -> ("Value"=w177:dbl)  [unwired: 2 in, 2 out]
                  n222 = property on="Ga Prep var" class="Bool (strict)"() -> ("Value"=w179:bool)  [unwired: 2 in, 2 out]
                  n223 = property on="Ga Run" class="Bool (strict)"() -> ("Value"=w180:bool)  [unwired: 2 in, 2 out]
                  n224 = And(x=w179, y=w180) -> (x .and. y?=w182:bool)
                  n225 = property on="Ga Dilution" class="Bool (strict)"() -> ("Value"=w181:bool)  [unwired: 2 in, 2 out]
                  n226 = call "set_Ga.vi"("Ga Active"=w178, "Ga Flow 3"=w175, "Ga Flow 2"=w176, "Ga Flow 1"=w177, "Ga Bubbler"=w178, "Ga H2 Dilute"=w181, "Ga Run"=w182, "Ga Remote"=w178) -> ()  [unwired: 8 in]
                }
              }
            }
            frame True {
            }
          }
        }
        frame #2 {
          n227 = case shown="False" w183 {
            frame False {
              n228 = property on="In?" class="Bool (strict)"() -> ("Value"=w184:bool)  [unwired: 2 in, 2 out]
              n229 = case shown="True" w184 {
                frame False {
                  w186 = FALSE ("In Remote")
                  n230 = call "set_In.vi"("Indium Flow"=0.0, "In Remote"=w186, "In Run"=w186, "In Bubbler"=w186, "In Active"=w186) -> ()  [unwired: 5 out]
                }
                frame True {
                  w191 = TRUE ("In Run")
                  n231 = property on="In Run" class="Bool (strict)"() -> ("Value"=w188:bool)  [unwired: 2 in, 2 out]
                  n232 = property on="In Prep" class="Bool (strict)"() -> ("Value"=w189:bool)  [unwired: 2 in, 2 out]
                  n233 = And(x=w189, y=w188) -> (x .and. y?=w187:bool)
                  n234 = property on="In Flow" class="DigNum (strict)"() -> ("Value"=w190:dbl)  [unwired: 2 in, 2 out]
                  n235 = call "set_In.vi"("Indium Flow"=w190, "In Run"=w187, "In Bubbler"=w191, "In Active"=w191) -> ()  [unwired: 1 in, 5 out]
                }
              }
            }
            frame True {
            }
          }
        }
        frame #3 {
          n236 = case shown="False" w192 {
            frame False {
              n237 = property on="PH3?" class="Bool (strict)"() -> ("Value"=w193:bool)  [unwired: 2 in, 2 out]
              n238 = case shown="True" w193 {
                frame False {
                  w194 = FALSE ("P_Gas Active")
                  n239 = call "set_P_gas.vi"("P_Gas Active"=w194, "P_Gas Flow"=0.0, "P_Gas In"=w194, "P_Gas H2 In"=w194, "P_Gas Run"=w194, "P_Gas Remote"=w194) -> ()  [unwired: 10 out]
                }
                frame True {
                  w200 = TRUE ("P_Gas Active")
                  n240 = property on="PH3 Flow" class="DigNum (strict)"() -> ("Value"=w199:dbl)  [unwired: 2 in, 2 out]
                  n241 = property on="PH3 Prep" class="Bool (strict)"() -> ("Value"=w198:bool)  [unwired: 2 in, 2 out]
                  n242 = property on="PH3 Run" class="Bool (strict)"() -> ("Value"=w197:bool)  [unwired: 2 in, 2 out]
                  n243 = And(x=w198, y=w197) -> (x .and. y?=w196:bool)
                  n244 = call "set_P_gas.vi"("P_Gas Active"=w200, "P_Gas Flow"=w199, "P_Gas In"=w200, "P_Gas Run"=w196) -> ()  [unwired: 2 in, 10 out]
                }
              }
            }
            frame True {
            }
          }
        }
        frame #4 {
          n245 = case shown="False" w201 {
            frame False {
              n246 = property on="AsH3?" class="Bool (strict)"() -> ("Value"=w202:bool)  [unwired: 2 in, 2 out]
              n247 = case shown="True" w202 {
                frame False {
                  w203 = FALSE ("As_Gas Active")
                  n248 = call "set_As_gas.vi"("As_Gas Active"=w203, "As_Gas Flow"=0.0, "As_Gas In"=w203, "As_Gas H2"=w203, "As_Gas Run"=w203, "As_Gas Remote"=w203) -> ()  [unwired: 10 in]
                }
                frame True {
                  w209 = TRUE ("As_Gas Active")
                  n249 = property on="AsH3 Prep" class="Bool (strict)"() -> ("Value"=w206:bool)  [unwired: 2 in, 2 out]
                  n250 = property on="AsH3 Run" class="Bool (strict)"() -> ("Value"=w207:bool)  [unwired: 2 in, 2 out]
                  n251 = property on="AsH3 Flow" class="DigNum (strict)"() -> ("Value"=w208:dbl)  [unwired: 2 in, 2 out]
                  n252 = And(x=w206, y=w207) -> (x .and. y?=w205:bool)
                  n253 = call "set_As_gas.vi"("As_Gas Active"=w209, "As_Gas Flow"=w208, "As_Gas In"=w209, "As_Gas Run"=w205) -> ()  [unwired: 12 in]
                }
              }
            }
            frame True {
            }
          }
        }
      }
    }
    frame "Run" {
      n254 = stacked-sequence {
        tunnel: w213 -> [_ w218 _ _]
        tunnel: w210 -> [w215 _ _ w281]
        tunnel: [_ _ _ w280] -> w212
        tunnel: w211 -> [_ _ _ w282]
        frame #0 {
          n255 = call "Get_Argument.vi"("Argument"="run_started", "Argument List"=w215) -> ("Enabled"=w214:bool)
          n256 = local write "run started"(w214) -> ()
        }
        frame #1 {
          n257 = property on="prep_time" class="DigNum (strict)"() -> ("Value"=w219:dbl)  [unwired: 2 in, 2 out]
          n258 = Greater Or Equal?(x=w218, y=w219) -> (x >= y?=w217:bool)
          n259 = local write "prep_done"(w217) -> ()
        }
        frame #2 {
          n260 = local read "run started"() -> (w221:bool)
          n261 = Not(x=w221) -> (.not. x?=w220:bool)
          n262 = stacked-sequence {
            tunnel: w220 -> [w223 w227 w236 w245 w254 w263 w274]
            frame #0 {
              n263 = case shown="True" w223 {
                tunnel: ["run: " "pre-run: "] -> w222
                frame False {
                }
                frame True {
                }
              }
              n264 = property on="Status Out" class="Str"("Value"=w222) -> ()  [unwired: 2 in, 2 out]
            }
            frame #1 {
              n265 = property on="Status Out" class="Str"() -> ("Value"=w233:string)  [unwired: 2 in, 2 out]
              n266 = property on="Al?" class="Bool (strict)"() -> ("Value"=w234:bool)  [unwired: 2 in, 2 out]
              n267 = property on="Al Run" class="Bool (strict)"() -> ("Value"=w226:bool)  [unwired: 2 in, 2 out]
              n268 = property on="Al Prep" class="Bool (strict)"() -> ("Value"=w228:bool)  [unwired: 2 in, 2 out]
              n269 = call "flow_strings.vi"("string in"=w233, "is first in?"=TRUE, "use source?"=w234, "name"="Al", "run source?"=w226, "prep source?"=w228, "is prep?"=w227) -> ("string out"=w232:string, "is first out?"=w231:bool)
              n270 = property on="Status Out" class="Str"("Value"=w232) -> ()  [unwired: 2 in, 2 out]
              n271 = property on="first" class="Bool (strict)"("Value"=w231) -> ()  [unwired: 2 in, 2 out]
            }
            frame #2 {
              n272 = property on="first" class="Bool (strict)"() -> ("Value"=w239:bool)  [unwired: 2 in, 2 out]
              n273 = property on="Status Out" class="Str"() -> ("Value"=w242:string)  [unwired: 2 in, 2 out]
              n274 = property on="Ga?" class="Bool (strict)"() -> ("Value"=w240:bool)  [unwired: 2 in, 2 out]
              n275 = property on="Ga Run" class="Bool (strict)"() -> ("Value"=w235:bool)  [unwired: 2 in, 2 out]
              n276 = property on="Ga Prep" class="Bool (strict)"() -> ("Value"=w237:bool)  [unwired: 2 in, 2 out]
              n277 = call "flow_strings.vi"("string in"=w242, "is first in?"=w239, "use source?"=w240, "name"="Ga", "run source?"=w235, "prep source?"=w237, "is prep?"=w236) -> ("string out"=w243:string, "is first out?"=w238:bool)
              n278 = property on="Status Out" class="Str"("Value"=w243) -> ()  [unwired: 2 in, 2 out]
              n279 = property on="first" class="Bool (strict)"("Value"=w238) -> ()  [unwired: 2 in, 2 out]
            }
            frame #3 {
              n280 = property on="first" class="Bool (strict)"() -> ("Value"=w249:bool)  [unwired: 2 in, 2 out]
              n281 = property on="Status Out" class="Str"() -> ("Value"=w251:string)  [unwired: 2 in, 2 out]
              n282 = property on="In?" class="Bool (strict)"() -> ("Value"=w252:bool)  [unwired: 2 in, 2 out]
              n283 = property on="In Run" class="Bool (strict)"() -> ("Value"=w244:bool)  [unwired: 2 in, 2 out]
              n284 = property on="In Prep" class="Bool (strict)"() -> ("Value"=w246:bool)  [unwired: 2 in, 2 out]
              n285 = call "flow_strings.vi"("string in"=w251, "is first in?"=w249, "use source?"=w252, "name"="In", "run source?"=w244, "prep source?"=w246, "is prep?"=w245) -> ("string out"=w248:string, "is first out?"=w247:bool)
              n286 = property on="Status Out" class="Str"("Value"=w248) -> ()  [unwired: 2 in, 2 out]
              n287 = property on="first" class="Bool (strict)"("Value"=w247) -> ()  [unwired: 2 in, 2 out]
            }
            frame #4 {
              n288 = property on="first" class="Bool (strict)"() -> ("Value"=w257:bool)  [unwired: 2 in, 2 out]
              n289 = property on="Status Out" class="Str"() -> ("Value"=w259:string)  [unwired: 2 in, 2 out]
              n290 = property on="PH3?" class="Bool (strict)"() -> ("Value"=w260:bool)  [unwired: 2 in, 2 out]
              n291 = property on="PH3 Run" class="Bool (strict)"() -> ("Value"=w253:bool)  [unwired: 2 in, 2 out]
              n292 = property on="PH3 Prep" class="Bool (strict)"() -> ("Value"=w255:bool)  [unwired: 2 in, 2 out]
              n293 = call "flow_strings.vi"("string in"=w259, "is first in?"=w257, "use source?"=w260, "name"="PH3", "run source?"=w253, "prep source?"=w255, "is prep?"=w254) -> ("string out"=w258:string, "is first out?"=w256:bool)
              n294 = property on="Status Out" class="Str"("Value"=w258) -> ()  [unwired: 2 in, 2 out]
              n295 = property on="first" class="Bool (strict)"("Value"=w256) -> ()  [unwired: 2 in, 2 out]
            }
            frame #5 {
              n296 = property on="first" class="Bool (strict)"() -> ("Value"=w266:bool)  [unwired: 2 in, 2 out]
              n297 = property on="Status Out" class="Str"() -> ("Value"=w268:string)  [unwired: 2 in, 2 out]
              n298 = property on="AsH3?" class="Bool (strict)"() -> ("Value"=w269:bool)  [unwired: 2 in, 2 out]
              n299 = property on="AsH3 Run" class="Bool (strict)"() -> ("Value"=w262:bool)  [unwired: 2 in, 2 out]
              n300 = property on="AsH3 Prep" class="Bool (strict)"() -> ("Value"=w264:bool)  [unwired: 2 in, 2 out]
              n301 = call "flow_strings.vi"("string in"=w268, "is first in?"=w266, "use source?"=w269, "name"="AsH3", "run source?"=w262, "prep source?"=w264, "is prep?"=w263) -> ("string out"=w265:string, "is first out?"=w267:bool)
              n302 = property on="Status Out" class="Str"("Value"=w265) -> ()  [unwired: 2 in, 2 out]
              n303 = property on="first" class="Bool (strict)"("Value"=w267) -> ()  [unwired: 2 in, 2 out]
            }
            frame #6 {
              n304 = property on="Pbub?" class="Bool (strict)"() -> ("Value"=w271:bool)  [unwired: 2 in, 2 out]
              n305 = property on="first" class="Bool (strict)"() -> ("Value"=w276:bool)  [unwired: 2 in, 2 out]
              n306 = property on="Status Out" class="Str"() -> ("Value"=w278:string)  [unwired: 2 in, 2 out]
              n307 = property on="Pbub Run" class="Bool (strict)"() -> ("Value"=w272:bool)  [unwired: 2 in, 2 out]
              n308 = property on="Pbub Prep" class="Bool (strict)"() -> ("Value"=w273:bool)  [unwired: 2 in, 2 out]
              n309 = call "flow_strings.vi"("string in"=w278, "is first in?"=w276, "use source?"=w271, "name"="Pbub", "run source?"=w272, "prep source?"=w273, "is prep?"=w274) -> ("string out"=w277:string, "is first out?"=w275:bool)
              n310 = property on="Status Out" class="Str"("Value"=w277) -> ()  [unwired: 2 in, 2 out]
              n311 = property on="first" class="Bool (strict)"("Value"=w275) -> ()  [unwired: 2 in, 2 out]
            }
          }
        }
        frame #3 {
          n312 = local read "run started"() -> (w285:bool)
          n313 = local read "prep_done"() -> (w283:bool)
          n314 = Not(x=w285) -> (.not. x?=w286:bool)
          n315 = And(x=w283, y=w286) -> (x .and. y?=w284:bool)
          n316 = stacked-sequence {
            tunnel: w284 -> [w290]
            tunnel: w282 -> [w289]
            tunnel: w281 -> [w288]
            tunnel: [w287] -> w280
            frame #0 {
              n317 = case shown="True" w290 {
                tunnel: w289 -> [_ w294]
                tunnel: w288 -> [w291 w293]
                tunnel: [w291 w292] -> w287
                frame False {
                }
                frame True {
                  n318 = stacked-sequence {
                    tunnel: w294 -> [w295 w302 w312 w319 w326 w333 _]
                    tunnel: w293 -> [_ _ _ _ _ _ w341]
                    tunnel: [_ _ _ _ _ _ w340] -> w292
                    frame #0 {
                      n319 = case shown="False" w295 {
                        frame False {
                          n320 = property on="Al?" class="Bool (strict)"() -> ("Value"=w296:bool)  [unwired: 2 in, 2 out]
                          n321 = case shown="True" w296 {
                            frame False {
                              w297 = FALSE ("Al Active")
                              n322 = call "set_Al.vi"("Aluminum Flow"=0.0, "Al Remote"=w297, "Al Run"=w297, "Al Bubbler"=w297, "Al Active"=w297) -> ()  [unwired: 5 out]
                            }
                            frame True {
                              w301 = TRUE ("Al Active")
                              n323 = property on="Al Flow" class="DigNum (strict)"() -> ("Value"=w300:dbl)  [unwired: 2 in, 2 out]
                              n324 = property on="Al Run" class="Bool (strict)"() -> ("Value"=w299:bool)  [unwired: 2 in, 2 out]
                              n325 = call "set_Al.vi"("Aluminum Flow"=w300, "Al Run"=w299, "Al Bubbler"=w301, "Al Active"=w301) -> ()  [unwired: 1 in, 5 out]
                            }
                          }
                        }
                        frame True {
                        }
                      }
                    }
                    frame #1 {
                      n326 = case shown="False" w302 {
                        frame False {
                          n327 = property on="Ga?" class="Bool (strict)"() -> ("Value"=w303:bool)  [unwired: 2 in, 2 out]
                          n328 = case shown="True" w303 {
                            frame False {
                              w305 = FALSE ("Ga Active")
                              w304 = 0.0 ("Ga Flow 1")
                              n329 = call "set_Ga.vi"("Ga Active"=w305, "Ga Flow 3"=w304, "Ga Flow 2"=w304, "Ga Flow 1"=w304, "Ga Bubbler"=w305, "Ga H2 Dilute"=w305, "Ga Run"=w305, "Ga Remote"=w305) -> ()  [unwired: 8 out]
                            }
                            frame True {
                              w310 = TRUE ("Ga Active")
                              n330 = property on="GAMFC3 var" class="DigNum (strict)"() -> ("Value"=w306:dbl)  [unwired: 2 in, 2 out]
                              n331 = property on="Ga Dilution" class="Bool (strict)"() -> ("Value"=w309:bool)  [unwired: 2 in, 2 out]
                              n332 = property on="Ga Run" class="Bool (strict)"() -> ("Value"=w311:bool)  [unwired: 2 in, 2 out]
                              n333 = property on="GAMFC2 var" class="DigNum (strict)"() -> ("Value"=w307:dbl)  [unwired: 2 in, 2 out]
                              n334 = property on="GAMFC1 var" class="DigNum (strict)"() -> ("Value"=w308:dbl)  [unwired: 2 in, 2 out]
                              n335 = call "set_Ga.vi"("Ga Active"=w310, "Ga Flow 3"=w306, "Ga Flow 2"=w307, "Ga Flow 1"=w308, "Ga Bubbler"=w310, "Ga H2 Dilute"=w309, "Ga Run"=w311, "Ga Remote"=w310) -> ()  [unwired: 8 in]
                            }
                          }
                        }
                        frame True {
                        }
                      }
                    }
                    frame #2 {
                      n336 = case shown="False" w312 {
                        frame False {
                          n337 = property on="In?" class="Bool (strict)"() -> ("Value"=w313:bool)  [unwired: 2 in, 2 out]
                          n338 = case shown="True" w313 {
                            frame False {
                              w315 = FALSE ("In Remote")
                              n339 = call "set_In.vi"("Indium Flow"=0.0, "In Remote"=w315, "In Run"=w315, "In Bubbler"=w315, "In Active"=w315) -> ()  [unwired: 5 out]
                            }
                            frame True {
                              w318 = TRUE ("In Run")
                              n340 = property on="In Run" class="Bool (strict)"() -> ("Value"=w316:bool)  [unwired: 2 in, 2 out]
                              n341 = property on="In Flow" class="DigNum (strict)"() -> ("Value"=w317:dbl)  [unwired: 2 in, 2 out]
                              n342 = call "set_In.vi"("Indium Flow"=w317, "In Run"=w316, "In Bubbler"=w318, "In Active"=w318) -> ()  [unwired: 1 in, 5 out]
                            }
                          }
                        }
                        frame True {
                        }
                      }
                    }
                    frame #3 {
                      n343 = case shown="False" w319 {
                        frame False {
                          n344 = property on="PH3?" class="Bool (strict)"() -> ("Value"=w320:bool)  [unwired: 2 in, 2 out]
                          n345 = case shown="True" w320 {
                            frame False {
                              w321 = FALSE ("P_Gas Active")
                              n346 = call "set_P_gas.vi"("P_Gas Active"=w321, "P_Gas Flow"=0.0, "P_Gas In"=w321, "P_Gas H2 In"=w321, "P_Gas Run"=w321, "P_Gas Remote"=w321) -> ()  [unwired: 10 out]
                            }
                            frame True {
                              w325 = TRUE ("P_Gas Active")
                              n347 = property on="PH3 Flow" class="DigNum (strict)"() -> ("Value"=w324:dbl)  [unwired: 2 in, 2 out]
                              n348 = property on="PH3 Run" class="Bool (strict)"() -> ("Value"=w323:bool)  [unwired: 2 in, 2 out]
                              n349 = call "set_P_gas.vi"("P_Gas Active"=w325, "P_Gas Flow"=w324, "P_Gas In"=w325, "P_Gas Run"=w323) -> ()  [unwired: 2 in, 10 out]
                            }
                          }
                        }
                        frame True {
                        }
                      }
                    }
                    frame #4 {
                      n350 = case shown="False" w326 {
                        frame False {
                          n351 = property on="AsH3?" class="Bool (strict)"() -> ("Value"=w327:bool)  [unwired: 2 in, 2 out]
                          n352 = case shown="True" w327 {
                            frame False {
                              w328 = FALSE ("As_Gas Active")
                              n353 = call "set_As_gas.vi"("As_Gas Active"=w328, "As_Gas Flow"=0.0, "As_Gas In"=w328, "As_Gas H2"=w328, "As_Gas Run"=w328, "As_Gas Remote"=w328) -> ()  [unwired: 10 in]
                            }
                            frame True {
                              w331 = TRUE ("As_Gas Active")
                              n354 = property on="AsH3 Run" class="Bool (strict)"() -> ("Value"=w330:bool)  [unwired: 2 in, 2 out]
                              n355 = property on="AsH3 Flow" class="DigNum (strict)"() -> ("Value"=w332:dbl)  [unwired: 2 in, 2 out]
                              n356 = call "set_As_gas.vi"("As_Gas Active"=w331, "As_Gas Flow"=w332, "As_Gas In"=w331, "As_Gas Run"=w330) -> ()  [unwired: 12 in]
                            }
                          }
                        }
                        frame True {
                        }
                      }
                    }
                    frame #5 {
                      n357 = case shown="False" w333 {
                        frame False {
                          n358 = property on="PH3?" class="Bool (strict)"() -> ("Value"=w334:bool)  [unwired: 2 in, 2 out]
                          n359 = case shown="False" w334 {
                            frame False {
                              w335 = FALSE ("P_Gas Active")
                              n360 = call "set_P_Liq.vi"("P_Liq Flow"=0.0 ("P_Gas Flow"), "P_Liq Remote"=w335, "P_Liq Run"=w335, "P_Liq Bubbler"=w335, "P_Liq Active"=w335) -> ()  [unwired: 7 in]
                            }
                            frame True {
                              w339 = TRUE ("P_Gas Active")
                              n361 = property on="Pbub Flow" class="DigNum (strict)"() -> ("Value"=w338:dbl)  [unwired: 2 in, 2 out]
                              n362 = property on="Pbub Run" class="Bool (strict)"() -> ("Value"=w337:bool)  [unwired: 2 in, 2 out]
                              n363 = call "set_P_Liq.vi"("P_Liq Flow"=w338, "P_Liq Run"=w337, "P_Liq Bubbler"=w339, "P_Liq Active"=w339) -> ()  [unwired: 8 in]
                            }
                          }
                        }
                        frame True {
                        }
                      }
                    }
                    frame #6 {
                      n364 = call "Set_Argument.vi"("Enable"=TRUE, "Argument"="run_started", "Argument List In"=w341) -> ("Argument List Out"=w340:string[])
                    }
                  }
                }
              }
            }
          }
        }
      }
    }
    frame "End" {
    }
    frame "Idle" {
    }
  }
  "Argument List Out" <- w10
